vi "Read TC_PWM.vi"(0 "read buffer":string, 11 "Error In":errorcluster) -> (4 "Temp (C)":dbl, 6 "On/Off Actual":bool, 8 "On/Off Set":bool, 10 "Temp Set Point (C)":i32, 14 "PWM":i32, 15 "Error Out":errorcluster)   [LabVIEW 2015]
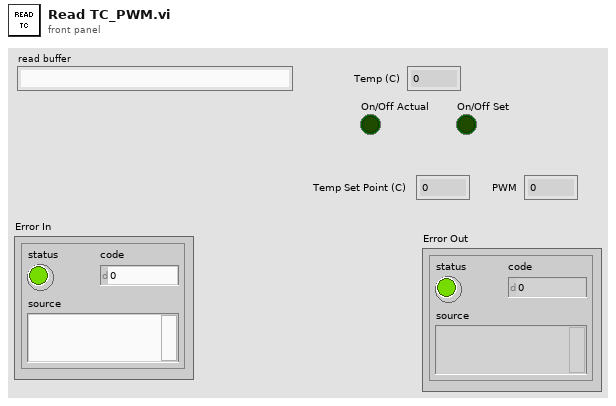
[diagram p1: front panel]
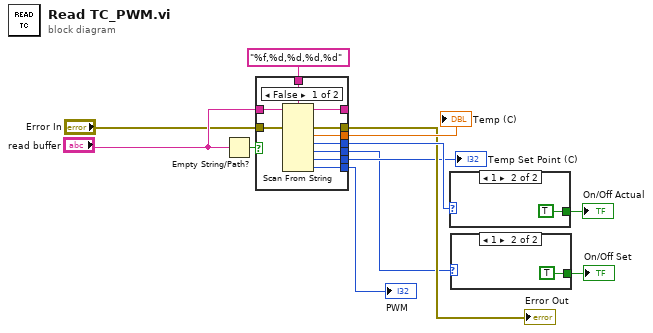
[diagram p0: block diagram]
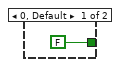
[diagram p2: hidden frame]
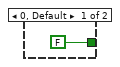
[diagram p3: hidden frame]
diagram:
  n1 = Empty String/Path?(string/path="read buffer") -> (empty?=w11:bool)
  n2 = case shown="False" w11 {
    tunnel: "read buffer" -> [w22 w24]
    tunnel: "%f,%d,%d,%d,%d" ("format string") -> [w21 _]
    tunnel: [w20 w24] -> _
    tunnel: [w19 _] -> w9
    tunnel: [w18 _] -> w2
    tunnel: [w17 _] -> w8
    tunnel: [w16 w23] -> w6
    tunnel: "Error In" -> [w15 w23]
    tunnel: [w14 _] -> w3
    tunnel: [w13 _] -> w1
    frame False {
      n3 = Scan From String(format string=w21, input string=w22, error in=w15) -> (remaining string=w20:string, error out=w16:errorcluster, output 1=w19:dbl, output 2=w17:i32, output 3=w18:i32, output 4=w14:i32, output 5=w13:i32)  [unwired: 6 in, 1 out]
    }
    frame True {
    }
  }
  "Temp (C)" <- w9
  "Temp Set Point (C)" <- w3
  "Error Out" <- w6
  "PWM" <- w1
  n4 = case shown="1" w8 {
    tunnel: [FALSE TRUE] -> w7
    frame 0, Default {
    }
    frame 1 {
    }
  }
  "On/Off Actual" <- w7
  n5 = case shown="1" w2 {
    tunnel: [FALSE TRUE] -> w4
    frame 0, Default {
    }
    frame 1 {
    }
  }
  "On/Off Set" <- w4
